vi "Read Module Decimation.vi"(7 "Module ID":string, 8 "error in":errorcluster, 11 "Standard Engine Repo Data in":refnum<class "Standard Engine Configuration.lvclass">) -> (0 "error out":errorcluster, 2 "Module Decimation":T1={"Decimation"=1, "Offset"=0}, 3 "Standard Engine Repo Data out":refnum<class "Standard Engine Configuration.lvclass">)   [LabVIEW 2013, in "Standard Engine Configuration.lvclass"]
doc: "Returns the decimation values for the specified module that were configured using the 'Write Module Decimation.vi'."
uses:
  Standard Engine Configuration.lvclass
  Module Decimation.ctl
  Standard Engine Configuration.lvclass/Standard Engine Configuration.ctl
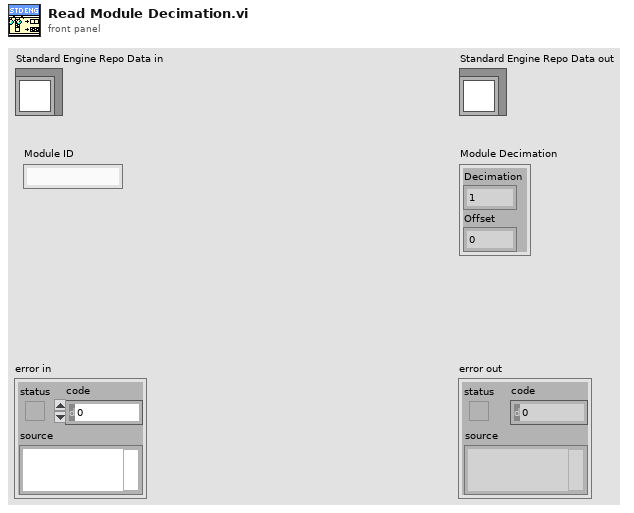
[diagram p1: front panel]
types:
  T1 = typedef "Standard Engine Configuration.lvclass/Module Decimation.ctl" = cluster{"Decimation":u16, "Offset":u16}
  T2 = typedef "Standard Engine Configuration.lvclass/Module Specific Configuration.ctl" = cluster{"Module ID":string, "Module Decimation":T1, "Module Error Configuration":T3, "execution order priority":i32, "async?":bool, "error tag":string}
  T3 = typedef "Standard Engine Configuration.lvclass/Module Error Configuration.ctl" = cluster{"Module Error Configuration":T4[]}
  T4 = typedef "Standard Engine Configuration.lvclass/Error Actions By Category.ctl" = cluster{"error classification":T5, "Error Actions":T6[]}
  T5 = typedef "TBM module execution interface.lvclass/error classification.ctl" = enum16{"unknown", "none", "trivial", "recoverable", "critical"}
  T6 = typedef "Standard Engine Configuration.lvclass/Error Actions.ctl" = enum16{"Clear", "Notify", "Stop Component", "Stop Engine", "Safe State", "Attempt Recovery"}
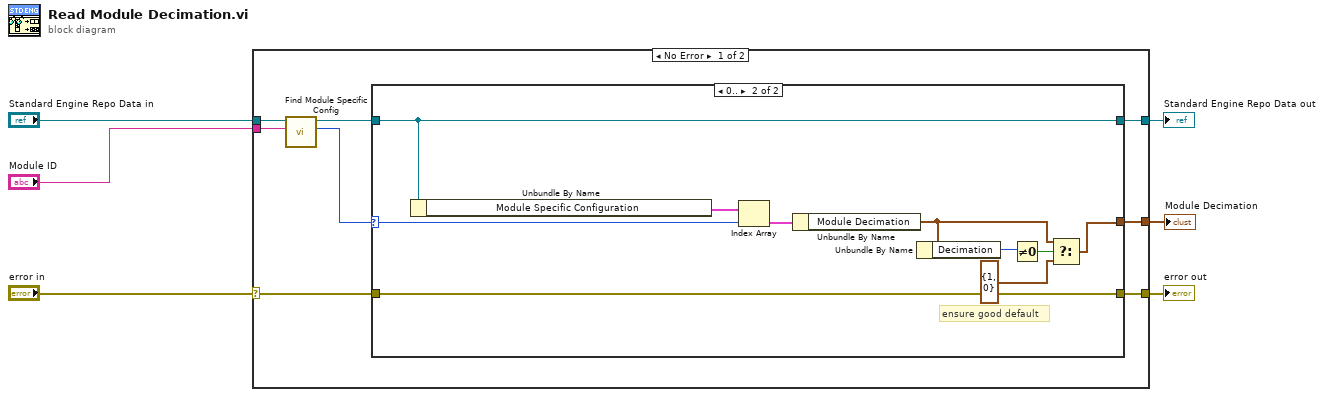
[diagram p0: block diagram]
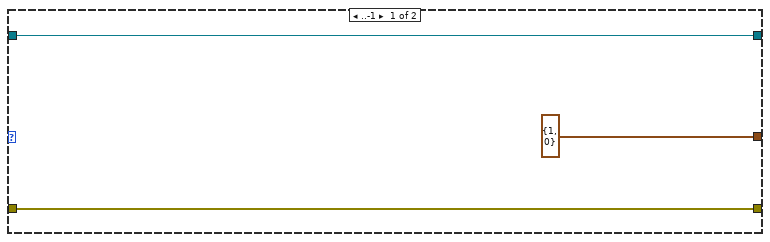
[diagram p2: hidden frame]
diagram:
  n1 = case shown="No Error" "error in" {
    selector: "error in" -> [w9 w29]
    tunnel: "Standard Engine Repo Data in" -> [w14 w28]
    tunnel: "Module ID" -> [w13 _]
    tunnel: [w7 w28] -> w4
    tunnel: [w11 _] -> w3
    tunnel: [w8 w29] -> w1
    frame No Error {
      n2 = call "Find Module Specific Config.vi"("Module ID"=w13, "Standard Engine Repo Data in"=w14) -> ("Index"=w10:i32, "Standard Engine Repo Data out"=w12:refnum<class "Standard Engine Configuration.lvclass">)  [unwired: 8 in]
      n3 = case shown="0.." w10 {
        selector: w10 -> [_ w24]
        tunnel: w12 -> [w17 w25]
        tunnel: [T1 {"Decimation"=1, "Offset"=0} ("Module Decimation") w19] -> w11
        tunnel: w9 -> [w16 w23]
        tunnel: [w16 w23] -> w8
        tunnel: [w17 w25] -> w7
        frame ..-1 {
        }
        frame 0.. {
          # "ensure good default"
          n4 = Unbundle By Name(w25) -> ("Module Specific Configuration"=w27:T2[])
          n5 = Index Array(array=w27, index=w24) -> (element=w26:T2)
          n6 = Unbundle By Name(w26) -> ("Module Decimation"=w20:T1)
          n7 = Unbundle By Name(w20) -> ("Decimation"=w22:u16)
          n8 = Not Equal To 0?(x=w22) -> (x != 0?=w21:bool)
          n9 = Select(t=w20, s=w21, f=T1 {"Decimation"=1, "Offset"=0} ("Module Decimation")) -> (s? t:f=w19:T1)
        }
      }
    }
    frame Error {
    }
  }
  "error out" <- w1
  "Standard Engine Repo Data out" <- w4
  "Module Decimation" <- w3
